vi "LinearPlntInvFF_New_Plant.vi"(6 "dT_Seconds":dbl=0.02, 11 "Plant":T1) -> (0 "Error":bool, 3 "Linear Plnt Inversion FF":T3)   [LabVIEW 2019, in "Trajectory_Library.lvlib"]
doc: "Constructs a plant inversion model-based feedforward from a LinearSystem.\n \nThe feedforward is calculated as \n\n u_ff = Binv (r_k+1 - A r_k) ,\n\nwhere \n\n Binv\n\nis the pseudoinverse of B.\n \nFor more on the underlying math, read https://file.tavsys.net/control/controls-engineering-in-frc.pdf.\n\nConstructs a feedforward with the given plant.\n \nInputs:\n - plant -- The plant being controlled.\n - dtSeconds -- Discretization timestep.\n\nOutputs:\n - outLinearPlntInversionFF -- updated system data cluster\n - error -- If TRUE, an error occured."
uses:
  Trajectory_Library.lvlib
  <vilib>/Analysis/Matrix/Datatypes/RealMatrix.ctl
  <vilib>/Analysis/Matrix/NI_Matrix.lvlib
  TypeDef/LINEAR_PLANT_INV_FF.ctl
  TypeDef/LINEAR_SYSTEM.ctl
panel:
  # "<States,States>"
  # "<States,Inputs>"
  # "<Outputs,States>"
  # "<Outputs,Inputs>"
  # "<States,1>"
  # "<Inputs,1>"
  # "<States,Inputs>"
  # "<States,States>"
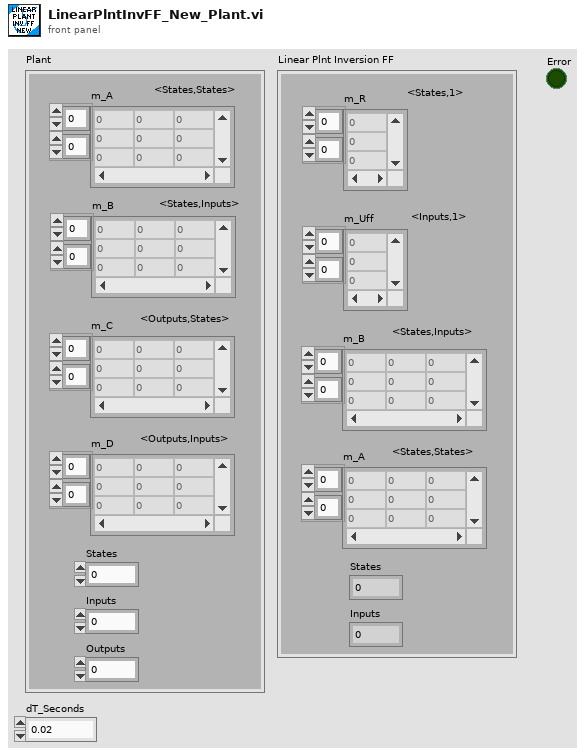
[diagram p1: front panel]
types:
  T1 = typedef "Trajectory_Library.lvlib/LINEAR_SYSTEM.ctl" = cluster{"m_A":T2, "m_B":T2, "m_C":T2, "m_D":T2, "States":i32, "Inputs":i32, "Outputs":i32}
  T2 = typedef "NI_Matrix.lvlib/RealMatrix.ctl" = dbl[][]
  T3 = typedef "Trajectory_Library.lvlib/LINEAR_PLANT_INV_FF.ctl" = cluster{"m_R":T2, "m_Uff":T2, "m_B":T2, "m_A":T2, "States":i32, "Inputs":i32}
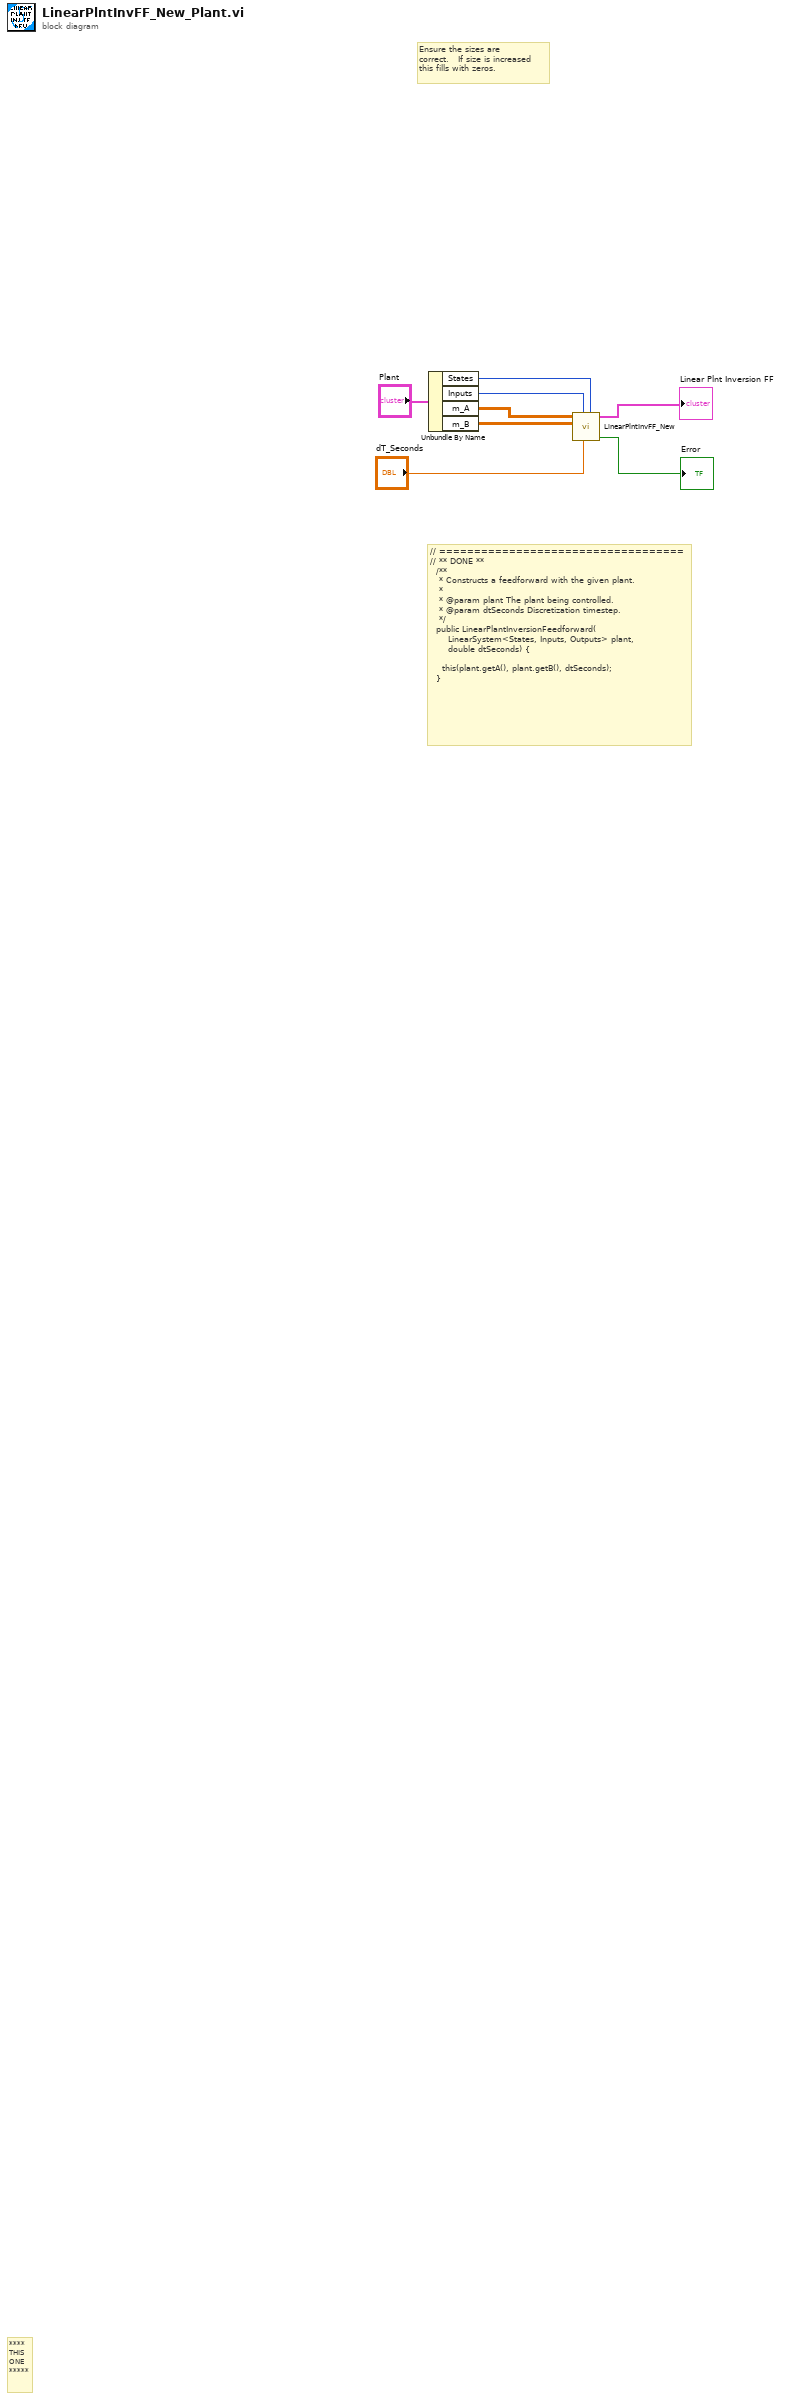
[diagram p0: block diagram]
diagram:
  # "// ===================================\n// ** DONE **\n  /**\n   * Constructs a feedforward with the given plant.\n   *\n   * @param plant The plant being controlled.\n   * @param dtSeconds Discretization timestep.\n   */\n  public LinearPlantInversionFeedforward(\n      LinearSystem<States, Inputs, Outputs> plant, \n      double dtSeconds) {\n\n    this(plant.getA(), plant.getB(), dtSeconds);\n  }"
  # "Ensure the sizes are\ncorrect.   If size is increased \nthis fills with zeros."
  # "****\nTHIS\nONE\n*****"
  n1 = Unbundle By Name("Plant") -> ("States"=w4:i32, "Inputs"=w5:i32, "m_A"=w7:T2, "m_B"=w6:T2)
  n2 = call "LinearPlntInvFF_New.vi"("States"=w4, "dT_Seconds"="dT_Seconds", "Inputs"=w5, "B"=w6, "A"=w7) -> ("Error"=→"Error":bool, "Linear Plnt Inversion FF"=→"Linear Plnt Inversion FF":T3)  [unwired: 5 in]
